vi "init_start_RBS.vi"(8 "error in (no error)":errorcluster) -> (0 "error out":errorcluster, 3 "RBS session out":T1)   [LabVIEW 2020]
uses:
  <vilib>/AKKA/PROVEtech-RBS/private/RBS Session.ctl
  <vilib>/AKKA/PROVEtech-RBS/private/RBS Core/RBS Core Data.ctl
  <vilib>/AKKA/PROVEtech-RBS/private/RBS status.ctl
  <vilib>/AKKA/PROVEtech-RBS/PROVEtechRBS.lvlib
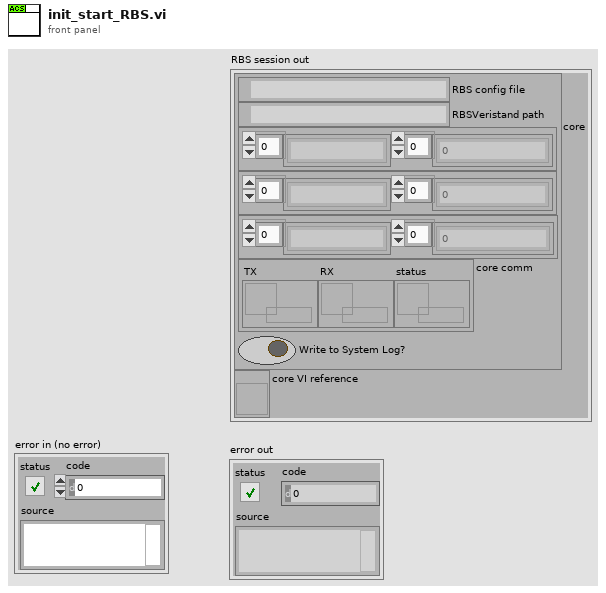
[diagram p1: front panel]
types:
  T1 = typedef "PROVEtechRBS.lvlib/RBS Session.ctl" = cluster{"core":T2, "core VI reference":refnum<vi>}
  T2 = typedef "PROVEtechRBS.lvlib/RBS Core Data.ctl" = cluster{"RBS config file":path, "RBSVeristand path":path, "TX signals":cluster{"names":string[], "values":dbl[]}, "RX signals":cluster{"names":string[], "values":dbl[]}, "TX_enable signals":cluster{"names":string[], "indices":i32[]}, "core comm":cluster{"TX":refnum<data-value>, "RX":refnum<data-value>, "status":refnum<data-value>}, "Write to System Log?":bool}
  T3 = typedef "PROVEtechRBS.lvlib/RBS Signal.ctl" = cluster{"Name":string, "Description":string, "Unit":string, "Lower Limit":dbl, "Upper Limit":dbl, "Signal Type":enum32{"RE_UINT8", "RE_INT8", "RE_UINT16", "RE_INT16", "RE_UINT32", "RE_INT32", "RE_UINT64", "RE_INT64", "RE_FLOAT32", "RE_FLOAT64"}, "ReadOnly":bool, "Signal Dimensions":i32[], "Default Value":dbl}
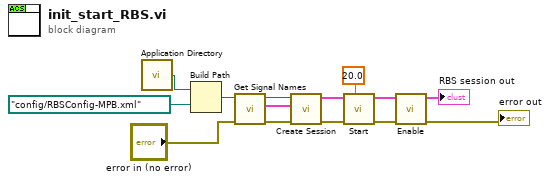
[diagram p0: block diagram]
diagram:
  n1 = call <vilib>:"Application Directory.vi"() -> ("Application Directory"=w6:path)
  n2 = Build Path(base path=w6, name or relative path=path "config/RBSConfig-MPB.xml") -> (appended path=w7:path)
  n3 = call <vilib>:"Get Signal Names.vi"("error in (no error)"="error in (no error)", "RBS config file in"=w7) -> ("error out"=w8:errorcluster, "RBS signal list"=w14:T3[], "RBS config file out"=w10:path)  [unwired: 7 in]
  n4 = call <vilib>:"Create Session.vi"("error in (no error)"=w8, "RBS signal list"=w14, "RBS Config File"=w10) -> ("error out"=w9:errorcluster, "RBS session out"=w11:T1)  [unwired: 5 in, 2 out]
  n5 = call <vilib>:"Start.vi"("timeout (10s)"=20.0, "error in (no error)"=w9, "RBS session in"=w11) -> ("error out"=w13:errorcluster, "RBS session out"=w12:T1)  [unwired: 7 in]
  n6 = call <vilib>:"Enable.vi"("error in (no error)"=w13, "RBS session in"=w12) -> ("error out"=→"error out":errorcluster, "RBS session out"=→"RBS session out":T1)  [unwired: 7 in, 1 out]
